vi "Variant Type to String Description.vi"(5 "Enum Names ?":bool, 7 "Include Names":bool, 8 "error in (no error)":errorcluster, 11 "Data Type":variant) -> (0 "error out":errorcluster, 2 "Top Level Type":string, 3 "String Representation of Type":string)   [LabVIEW 2012, in "Scripting Tools.lvlib" / "XNode Support.lvlib"]
doc: "Constructs a string that describes the type of data that has been wired to <b>Data Type</b>. Clusters and Arrays are recursively interpreted so that their elements type strings are embedded in the final <b>String Representation of Type</b>. For such compund types, the <b>Top Level Type<b> described the first level of the recursive type string. <b>Include Names</b> and <b>Enum Names</b> control whether the type string includes the cluster or array element names and whether enums contain a list of the possible enum labels.\n\nThis routine is designed to help test whether a particular XNode terminal type matches a string pattern."
uses:
  XNode Support.lvlib
  <vilib>/Utility/VariantDataType/Type.ctl
  <vilib>/Utility/VariantDataType/VariantType.lvlib
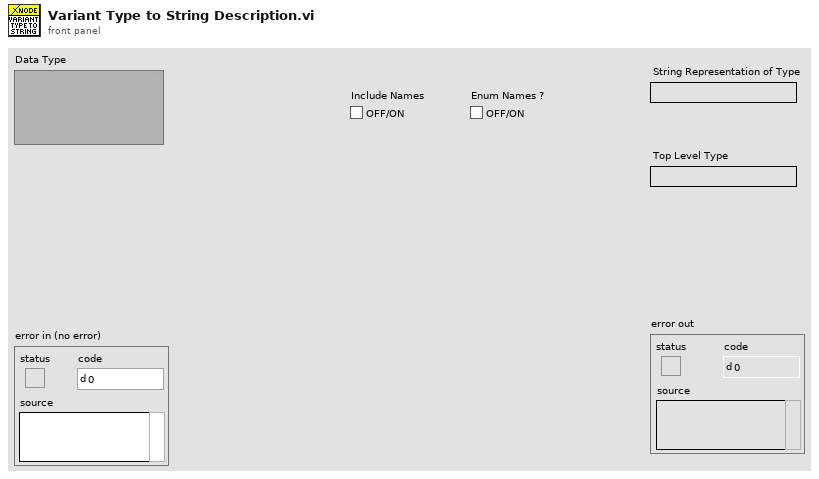
[diagram p1: front panel]
types:
  T1 = typedef "VariantType.lvlib/Type.ctl" = enum8{"Invalid Type", "Void", "I8", "I16", "I32", "I64", "U8", "U16", "U32", "U64", "Single Float", "Double Float", "Extended Float", "Single Complex", "Double Complex", "Extended Complex", "Enum U8", "Enum U16", "Enum U32", "Enum U64", "Single Float With Unit", "Double Float With Unit", "Extended Float With Unit", "Single Complex with Unit", "Double Complex with Unit", "Extended Complex with Unit", "Boolean", "String", "Path", "Picture", "Tag", "Array", "Cluster", "Variant", "LV Variant", "Waveform", "Timestamp", "Digital Waveform", "Digital Data", "ExpressData", "Refnum", "External Data", "VI", "Poly VI", "LabVIEW Class Instance", "Fixed Point"}
  T2 = typedef "VariantType.lvlib/RefnumType.ctl" = enum16{"NotARefnum", "UnknownRefnum", "Generic", "Datalog", "ByteStream", "Device", "Occurence", "TCPNetConnection", "Auto", "Menu", "Imaq", "Hardware", "DataSocket", "Visa", "IVI", "UDPNetConnection", "Notifier", "Queue", "Irda", "EventReg", "DotNet", "UserEvent", "Callback", "UNUSED_EMPTY_POSITION", "BlueToothNetConnection", "LVObjApp", "LVObjVI", "LVObjUnknown", "GenericClass", "UserDefinedRefnumTag", "DataValue", "RT FIFO", "TDMS File"}
  T3 = typedef "VariantType.lvlib/MemoryInfo.ctl" = cluster{"Type":T4, "Size":u32}
  T4 = typedef "VariantType.lvlib/MemoryType.ctl" = enum16{"Variable", "Fixed", "Bounded"}
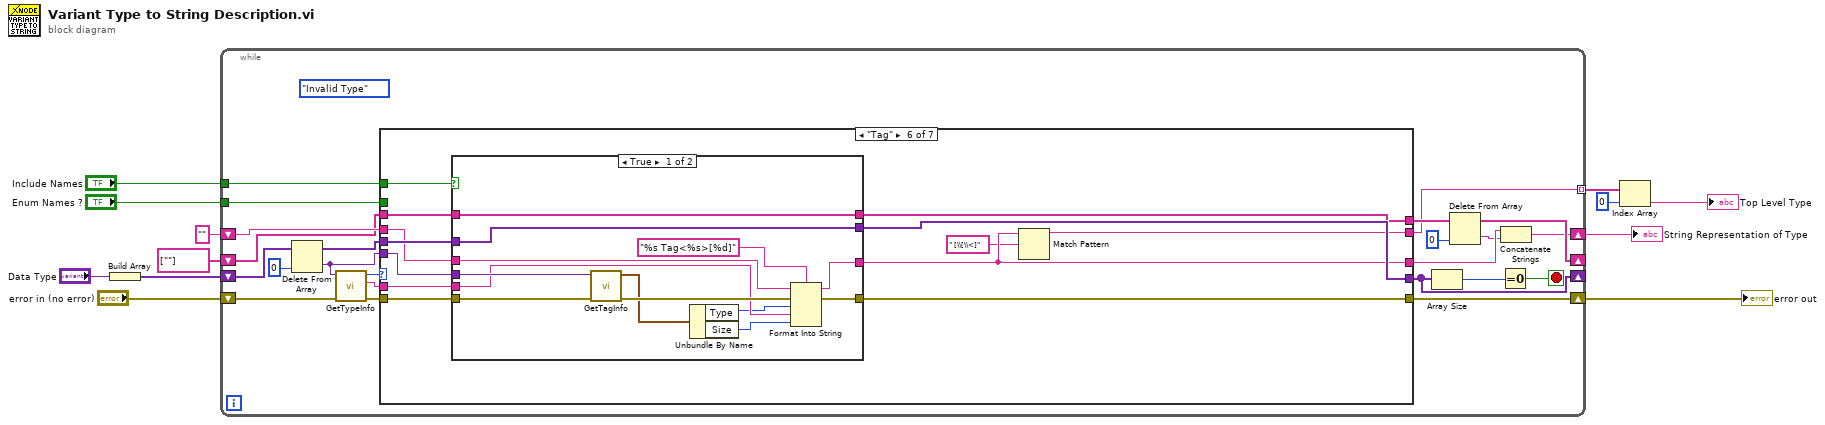
[diagram p0: block diagram]
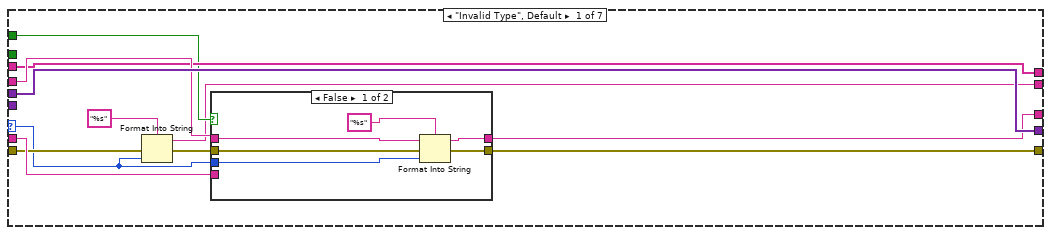
[diagram p2: hidden frame]
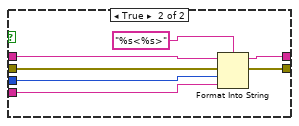
[diagram p3: hidden frame]
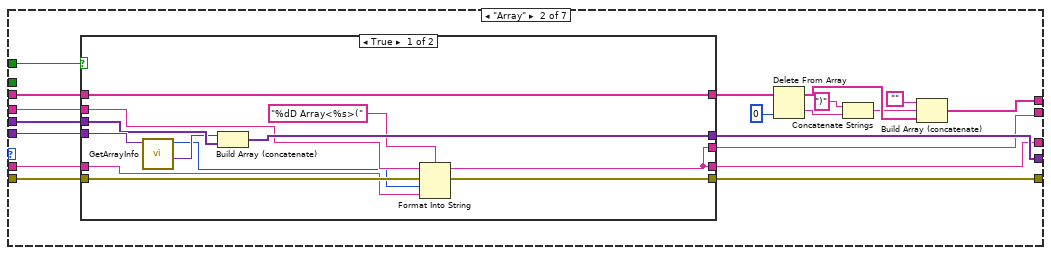
[diagram p4: hidden frame]
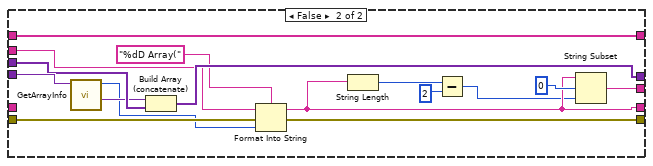
[diagram p5: hidden frame]
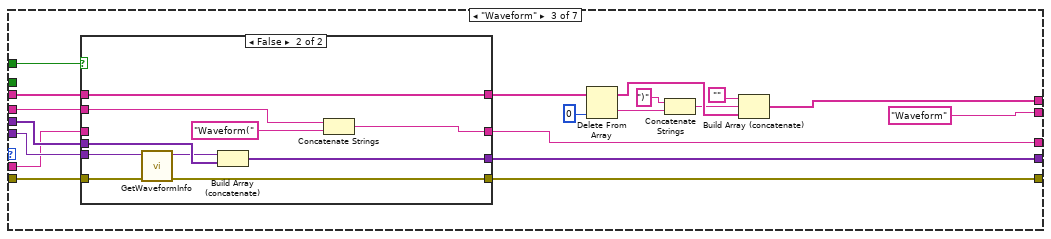
[diagram p6: hidden frame]
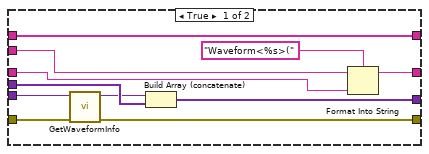
[diagram p7: hidden frame]
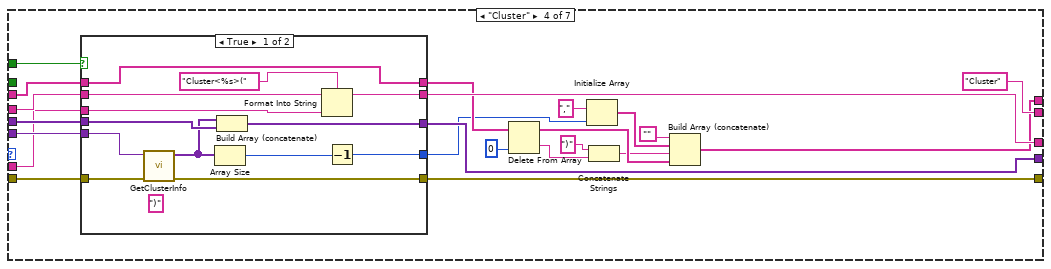
[diagram p8: hidden frame]
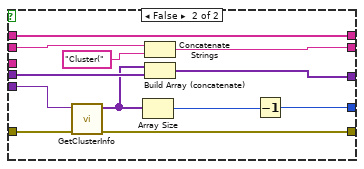
[diagram p9: hidden frame]
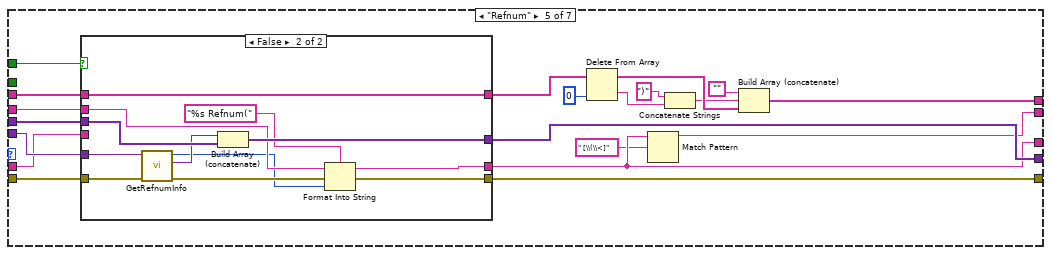
[diagram p10: hidden frame]
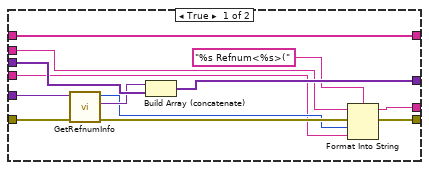
[diagram p11: hidden frame]
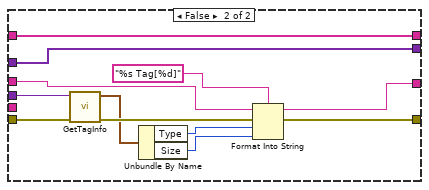
[diagram p12: hidden frame]
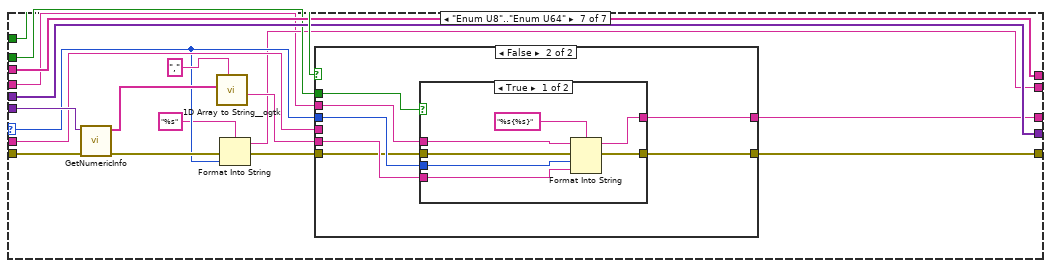
[diagram p13: hidden frame]
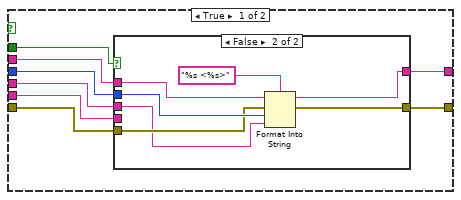
[diagram p14: hidden frame]
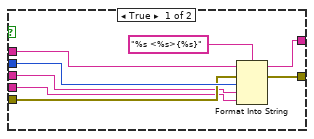
[diagram p15: hidden frame]
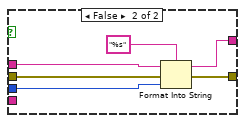
[diagram p16: hidden frame]
diagram:
  n1 = Build Array("Data Type") -> (w12:variant[])
  n2 = while {
    shift-right: [w28] -> _
    shift-left: w12 -> [w35]
    shift-right: [w24] -> w3
    shift-left: "error in (no error)" -> [w31]
    shift-right: [w16] -> w7
    shift-left: "" -> [w27]
    shift-right: [w18] -> _
    shift-left: string[] [""] -> [w14]
    tunnel: "Include Names" -> [w22]
    tunnel: "Enum Names ?" -> [w21]
    tunnel: [w19] -> w5 mode=indexing
    stop <- w33 stop-if-true
    (unwired) Type."Invalid Type" ("Type Enum")
    n3 = Delete From Array(array=w35, index=0) -> (deleted portion=w30:variant, array with subset deleted=w29:variant[])  [unwired: 1 in]
    n4 = call <vilib>:"GetTypeInfo.vi"("error in (no error)"=w31, "Variant"=w30) -> ("error out"=w25:errorcluster, "Name"=w32:string, "Type Enum"=w20:T1)  [unwired: 7 out]
    n5 = case shown="\"Tag\"" w20 {
      selector: w20 -> [w37 _ _ _ _ _ w281]
      tunnel: w32 -> [w41 w69 w118 w160 w207 w244 w285]
      tunnel: w30 -> [_ w79 w123 w167 w212 w250 w295]
      tunnel: w29 -> [w47 w78 w126 w169 w214 w252 w288]
      tunnel: [w47 w77 w125 w168 w213 w251 w288] -> w28
      tunnel: w27 -> [w46 w76 w120 w165 w210 w248 w278]
      tunnel: [w45 w73 w119 w164 w205 w242 w287] -> w26
      tunnel: w25 -> [w38 w75 w122 w166 w211 w249 w294]
      tunnel: [w44 w74 w121 w163 w209 w247 w289] -> w24
      tunnel: w14 -> [w43 w72 w124 w162 w208 w246 w286]
      tunnel: [w43 w63 w108 w153 w195 w245 w286] -> w23
      tunnel: w22 -> [w42 w70 w117 w161 w206 w243 w290]
      tunnel: w21 -> [_ _ _ _ _ _ w284]
      tunnel: [w36 w68 "Waveform" "Cluster" w203 w240 w279] -> w19
      frame "Invalid Type", Default {
        n6 = Format Into String(format string="%s", error in=w38, w37) -> (resulting string=w36:string, error out=w39:errorcluster)  [unwired: 1 in]
        n7 = case shown="False" w42 {
          tunnel: w46 -> [w53 w60]
          tunnel: w37 -> [w51 w58]
          tunnel: [w50 w57] -> w45
          tunnel: w39 -> [w49 w56]
          tunnel: [w48 w55] -> w44
          tunnel: w41 -> [_ w54]
          frame False {
            n8 = Format Into String(format string="%s", initial string=w53, error in=w49, w51) -> (resulting string=w50:string, error out=w48:errorcluster)
          }
          frame True {
            n9 = Format Into String(format string="%s<%s>", initial string=w60, error in=w56, w58, w54) -> (resulting string=w57:string, error out=w55:errorcluster)
          }
        }
      }
      frame "Array" {
        n10 = case shown="True" w70 {
          tunnel: w79 -> [w91 w107]
          tunnel: w78 -> [w90 w106]
          tunnel: [w88 w104] -> w77
          tunnel: w76 -> [w86 w103]
          tunnel: w75 -> [w85 w102]
          tunnel: [w84 w101] -> w74
          tunnel: [w80 w97] -> w73
          tunnel: w72 -> [w81 w92]
          tunnel: [w81 w92] -> w71
          tunnel: w69 -> [w82 _]
          tunnel: [w80 w93] -> w68
          frame True {
            n11 = call <vilib>:"GetArrayInfo.vi"("Variant"=w91) -> ("ArrayElement"=w89:variant, "NDims"=w83:i32)  [unwired: 1 in, 8 out]
            n12 = Build Array (concatenate)(w89, w90) -> (w88:variant[])
            n13 = Format Into String(format string="%dD Array<%s>(", initial string=w86, error in=w85, w83, w82) -> (resulting string=w80:string, error out=w84:errorcluster)
          }
          frame False {
            n14 = call <vilib>:"GetArrayInfo.vi"("Variant"=w107) -> ("ArrayElement"=w105:variant, "NDims"=w100:i32)  [unwired: 1 in, 8 out]
            n15 = Build Array (concatenate)(w105, w106) -> (w104:variant[])
            n16 = Format Into String(format string="%dD Array(", initial string=w103, error in=w102, w100) -> (resulting string=w97:string, error out=w101:errorcluster)
            n17 = String Length(string=w97) -> (length=w96:i32)
            n18 = Subtract(x=w96, y=2) -> (x-y=w94:i32)
            n19 = String Subset(string=w97, offset (0)=0, length (rest)=w94) -> (substring=w93:string)
          }
        }
        n20 = Delete From Array(array=w71, index=0) -> (deleted portion=w61:string, array with subset deleted=w64:string[])  [unwired: 1 in]
        n21 = Concatenate Strings(")", w61) -> (w62:string)
        n22 = Build Array (concatenate)("", w62, w64) -> (w63:string[])
      }
      frame "Waveform" {
        n23 = case shown="False" w117 {
          tunnel: w126 -> [w137 w147]
          tunnel: [w136 w146] -> w125
          tunnel: w124 -> [w127 w138]
          tunnel: [w127 w138] -> w109
          tunnel: w123 -> [w135 w145]
          tunnel: w122 -> [w133 w143]
          tunnel: [w132 w142] -> w121
          tunnel: w120 -> [w131 w141]
          tunnel: [w130 w140] -> w119
          tunnel: w118 -> [w128 _]
          frame True {
            n24 = call <vilib>:"GetWaveformInfo.vi"("error in (no error)"=w133, "Variant"=w135) -> ("error out"=w132:errorcluster, "YArrayType"=w134:variant)  [unwired: 8 out]
            n25 = Build Array (concatenate)(w134, w137) -> (w136:variant[])
            n26 = Format Into String(format string="Waveform<%s>(" ("string"), initial string=w131, w128) -> (resulting string=w130:string)  [unwired: 1 in, 1 out]
          }
          frame False {
            n27 = call <vilib>:"GetWaveformInfo.vi"("error in (no error)"=w143, "Variant"=w145) -> ("error out"=w142:errorcluster, "YArrayType"=w144:variant)  [unwired: 8 out]
            n28 = Build Array (concatenate)(w144, w147) -> (w146:variant[])
            n29 = Concatenate Strings(w141, "Waveform(" ("string")) -> (w140:string)
          }
        }
        n30 = Delete From Array(array=w109, index=0) -> (deleted portion=w110:string, array with subset deleted=w112:string[])  [unwired: 1 in]
        n31 = Concatenate Strings(")", w110) -> (w111:string)
        n32 = Build Array (concatenate)("", w111, w112) -> (w108:string[])
      }
      frame "Cluster" {
        n33 = case shown="True" w161 {
          tunnel: w169 -> [w182 w194]
          tunnel: [w181 w193] -> w168
          tunnel: w167 -> [w180 w192]
          tunnel: w166 -> [w179 w191]
          tunnel: w165 -> [w175 w190]
          tunnel: [w174 w189] -> w164
          tunnel: [w178 w188] -> w163
          tunnel: w162 -> [w171 w184]
          tunnel: w160 -> [w172 _]
          tunnel: [w171 w184] -> w158
          tunnel: [w170 w183] -> w156
          frame True {
            (unwired) ")"
            n34 = call <vilib>:"GetClusterInfo.vi"("error in (no error)"=w179, "Variant"=w180) -> ("error out"=w178:errorcluster, "Cluster Elements"=w177:variant[])  [unwired: 8 out]
            n35 = Array Size(array=w177) -> (size(s)=w176:i32)
            n36 = Build Array (concatenate)(w177, w182) -> (w181:variant[])
            n37 = Format Into String(format string="Cluster<%s>(" ("string"), initial string=w175, w172) -> (resulting string=w174:string)  [unwired: 1 in, 1 out]
            n38 = Decrement(x=w176) -> (x-1=w170:i32)
          }
          frame False {
            n39 = call <vilib>:"GetClusterInfo.vi"("error in (no error)"=w191, "Variant"=w192) -> ("error out"=w188:errorcluster, "Cluster Elements"=w186:variant[])  [unwired: 8 out]
            n40 = Array Size(array=w186) -> (size(s)=w185:i32)
            n41 = Concatenate Strings(w190, "Cluster(" ("string")) -> (w189:string)
            n42 = Build Array (concatenate)(w186, w194) -> (w193:variant[])
            n43 = Decrement(x=w185) -> (x-1=w183:i32)
          }
        }
        n44 = Delete From Array(array=w158, index=0) -> (deleted portion=w148:string, array with subset deleted=w152:string[])  [unwired: 1 in]
        n45 = Initialize Array(",", w156) -> (w155:string[])
        n46 = Concatenate Strings(")", w148) -> (w150:string)
        n47 = Build Array (concatenate)("", w155, w150, w152) -> (w153:string[])
      }
      frame "Refnum" {
        n48 = case shown="False" w206 {
          tunnel: w214 -> [w227 w239]
          tunnel: [w226 w238] -> w213
          tunnel: w212 -> [w225 w237]
          tunnel: w211 -> [w223 w235]
          tunnel: w210 -> [w221 w233]
          tunnel: [w220 w232] -> w205
          tunnel: [w218 w230] -> w209
          tunnel: w208 -> [w215 w228]
          tunnel: [w215 w228] -> w196
          tunnel: w207 -> [w216 _]
          frame True {
            n49 = call <vilib>:"GetRefnumInfo.vi"("error in (no error)"=w223, "Variant"=w225) -> ("error out"=w219:errorcluster, "StrictType"=w224:variant, "ReferenceType"=w217:T2)  [unwired: 7 out]
            n50 = Build Array (concatenate)(w224, w227) -> (w226:variant[])
            n51 = Format Into String(format string="%s Refnum<%s>(", initial string=w221, error in=w219, w217, w216) -> (resulting string=w220:string, error out=w218:errorcluster)
          }
          frame False {
            n52 = call <vilib>:"GetRefnumInfo.vi"("error in (no error)"=w235, "Variant"=w237) -> ("error out"=w231:errorcluster, "StrictType"=w236:variant, "ReferenceType"=w229:T2)  [unwired: 7 out]
            n53 = Build Array (concatenate)(w236, w239) -> (w238:variant[])
            n54 = Format Into String(format string="%s Refnum(", initial string=w233, error in=w231, w229) -> (resulting string=w232:string, error out=w230:errorcluster)
          }
        }
        n55 = Delete From Array(array=w196, index=0) -> (deleted portion=w197:string, array with subset deleted=w199:string[])  [unwired: 1 in]
        n56 = Match Pattern(string=w205, regular expression=" [\\(\\<]") -> (before substring=w203:string)  [unwired: 1 in, 3 out]
        n57 = Concatenate Strings(")", w197) -> (w198:string)
        n58 = Build Array (concatenate)("", w198, w199) -> (w195:string[])
      }
      frame "Tag" {
        n59 = case shown="True" w243 {
          tunnel: w252 -> [w257 w270]
          tunnel: [w257 w270] -> w251
          tunnel: w250 -> [w265 w277]
          tunnel: w249 -> [w264 w276]
          tunnel: w248 -> [w262 w274]
          tunnel: [w261 w273] -> w242
          tunnel: [w259 w271] -> w247
          tunnel: w246 -> [w253 w268]
          tunnel: [w253 w268] -> w245
          tunnel: w244 -> [w258 _]
          frame True {
            n60 = call <vilib>:"GetTagInfo.vi"("error in (no error)"=w264, "Variant"=w265) -> ("error out"=w260:errorcluster, "MemoryInfo"=w256:T3)  [unwired: 8 out]
            n61 = Unbundle By Name(w256) -> ("Type"=w254:T4, "Size"=w255:u32)
            n62 = Format Into String(format string="%s Tag<%s>[%d]", initial string=w262, error in=w260, w254, w258, w255) -> (resulting string=w261:string, error out=w259:errorcluster)
          }
          frame False {
            n63 = call <vilib>:"GetTagInfo.vi"("error in (no error)"=w276, "Variant"=w277) -> ("error out"=w272:errorcluster, "MemoryInfo"=w269:T3)  [unwired: 8 out]
            n64 = Unbundle By Name(w269) -> ("Type"=w266:T4, "Size"=w267:u32)
            n65 = Format Into String(format string="%s Tag[%d]", initial string=w274, error in=w272, w266, w267) -> (resulting string=w273:string, error out=w271:errorcluster)
          }
        }
        n66 = Match Pattern(string=w242, regular expression=" [\\[\\<]") -> (before substring=w240:string)  [unwired: 1 in, 3 out]
      }
      frame "Enum U8".."Enum U64" {
        n67 = call <vilib>:"GetNumericInfo.vi"("error in (no error)"=w294, "Variant"=w295) -> ("error out"=w283:errorcluster, "EnumNames"=w292:string[])  [unwired: 8 out]
        n68 = call <userlib>:"1D Array to String__ogtk.vi"("delimiter (Tab)"=",", "Array of Strings"=w292) -> ("delimited string"=w291:string)  [unwired: 9 out]
        n69 = Format Into String(format string="%s", error in=w283, w281) -> (resulting string=w279:string, error out=w282:errorcluster)  [unwired: 1 in]
        n70 = case shown="False" w290 {
          tunnel: w281 -> [w303 w325]
          tunnel: w291 -> [w299 w324]
          tunnel: w282 -> [w302 w323]
          tunnel: [w301 w322] -> w289
          tunnel: [w300 w321] -> w287
          tunnel: w285 -> [w298 _]
          tunnel: w284 -> [w297 w320]
          tunnel: w278 -> [w296 w319]
          frame True {
            n71 = case shown="False" w297 {
              tunnel: w303 -> [w310 w317]
              tunnel: w302 -> [w309 w316]
              tunnel: [w308 w315] -> w301
              tunnel: [w307 w314] -> w300
              tunnel: w299 -> [w306 _]
              tunnel: w298 -> [w305 w313]
              tunnel: w296 -> [w304 w312]
              frame True {
                n72 = Format Into String(format string="%s <%s>{%s}", initial string=w304, error in=w309, w310, w305, w306) -> (resulting string=w307:string, error out=w308:errorcluster)
              }
              frame False {
                n73 = Format Into String(format string="%s <%s>", initial string=w312, error in=w316, w317, w313) -> (resulting string=w314:string, error out=w315:errorcluster)
              }
            }
          }
          frame False {
            n74 = case shown="True" w320 {
              tunnel: w325 -> [w331 w337]
              tunnel: w324 -> [w330 _]
              tunnel: w323 -> [w329 w336]
              tunnel: [w328 w335] -> w322
              tunnel: [w327 w334] -> w321
              tunnel: w319 -> [w326 w333]
              frame True {
                n75 = Format Into String(format string="%s{%s}", initial string=w326, error in=w329, w331, w330) -> (resulting string=w327:string, error out=w328:errorcluster)
              }
              frame False {
                n76 = Format Into String(format string="%s", initial string=w333, error in=w336, w337) -> (resulting string=w334:string, error out=w335:errorcluster)
              }
            }
          }
        }
      }
    }
    n77 = Array Size(array=w28) -> (size(s)=w34:i32)
    n78 = Delete From Array(array=w23, index=0) -> (deleted portion=w15:string, array with subset deleted=w18:string[])  [unwired: 1 in]
    n79 = Equal To 0?(x=w34) -> (x = 0?=w33:bool)
    n80 = Concatenate Strings(w26, w15) -> (w16:string)
  }
  "error out" <- w3
  "String Representation of Type" <- w7
  n81 = Index Array(array=w5, index=0) -> (element=→"Top Level Type":string)
